vi "HelpMessage.vi"(11 "ExecuteAllBuildSpecs in":refnum<class "ExecuteAllBuildSpecs.lvclass">) -> (2 "Help":string, 3 "ExecuteAllBuildSpecs out":refnum<class "ExecuteAllBuildSpecs.lvclass">)   [LabVIEW 2014, in "ExecuteAllBuildSpecs.lvclass"]
doc: "The help message for this multiple build spec operation in the LabVIEWCLI."
uses:
  ExecuteAllBuildSpecs.lvclass
panel:
  in  "HelpText":string="LabVIEWCLI -OperationName ExecuteAllBuildSpecs -ProjectPath <path of LabVIEW project>\n\n -ProjectPath : Specifies the full path to the LabVIEW project (.lvproj) file that contains the build specifications.  All build specifications contained in this project will be built.\n"
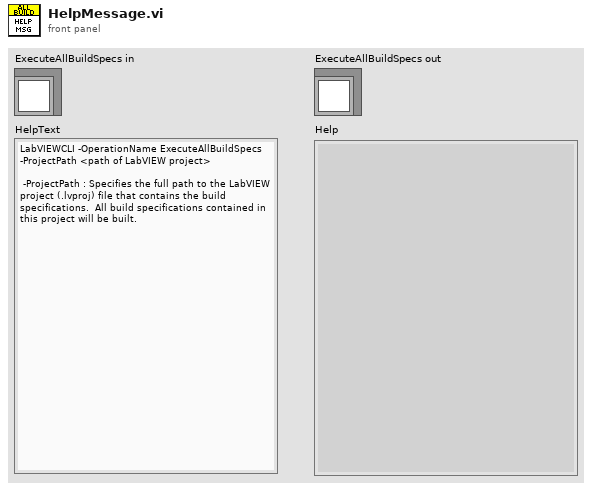
[diagram p1: front panel]
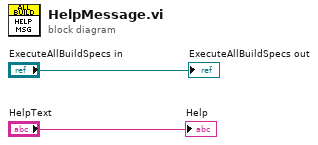
[diagram p0: block diagram]
diagram:
  "ExecuteAllBuildSpecs out" <- "ExecuteAllBuildSpecs in"
  "Help" <- "HelpText"
